vi "status of power_supply4.vi"() -> ()   [LabVIEW 2020]
panel:
  out "status of power_supply4":bool
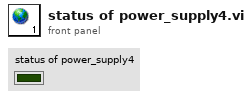
[diagram p1: front panel]
diagram:
